vi "Exp Inverse CDF.vi"(9 "b":dbl=3.0, 10 "a":dbl=1.0, 11 "cdf(x)":dbl=0.486583) -> (0 "error":i32, 3 "x":dbl=3.000000695531575)   [LabVIEW 2020, in "NI_Gmath.lvlib"]
doc: "Computes the continuous inverse cumulative distribution function (CDF) of the various distributions. You must manually select the polymorphic instance to use."
uses:
  <vilib>/gmath/NI_Gmath.lvlib
  <vilib>/gmath/statdist.llb/st_error_code.ctl
panel:
  # "Exp Inverse CDF"
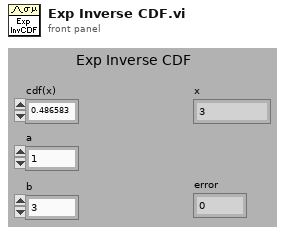
[diagram p1: front panel]
types:
  T1 = typedef "NI_Gmath.lvlib/st_error_code.ctl" = i32
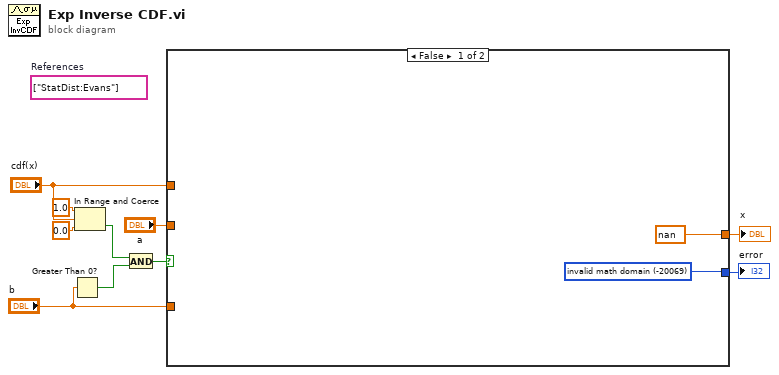
[diagram p0: block diagram]
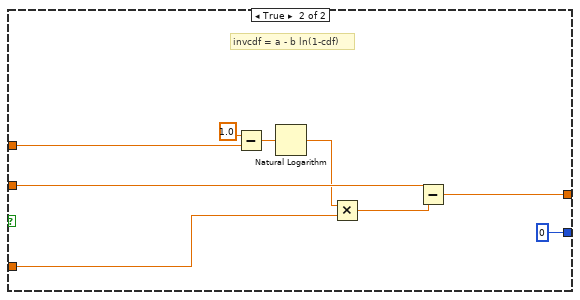
[diagram p2: hidden frame]
diagram:
  (unwired) string[] ["StatDist:Evans"]  # References
  n1 = Greater Than 0?(x="b") -> (x > 0?=w2:bool)
  n2 = In Range and Coerce(upper limit=1.0, x="cdf(x)", lower limit=0.0) -> (In Range?=w1:bool)  [unwired: 1 out]
  n3 = And(x=w1, y=w2) -> (x .and. y?=w3:bool)
  n4 = case shown="False" w3 {
    tunnel: "b" -> [_ w18]
    tunnel: [w11 0 ("invalid math domain")] -> w9
    tunnel: [nan w20] -> w8
    tunnel: "cdf(x)" -> [_ w17]
    tunnel: "a" -> [_ w19]
    frame False {
      w11 = T1 -20069 items=["invalid math domain"=-20069, "Fourier interpolation size m >= n"=-20070, "empty array"=-20003] ("stat interp error code")
    }
    frame True {
      # "invcdf = a - b ln(1-cdf)"
      n5 = Subtract(x=1.0 ("y"), y=w17) -> (x-y=w15:dbl)
      n6 = Natural Logarithm(1:w15) -> (0:w13:dbl)
      n7 = Multiply(x=w13, y=w18) -> (x*y=w14:dbl)
      n8 = Subtract(x=w19, y=w14) -> (x-y=w20:dbl)
    }
  }
  "x" <- w8
  "error" <- w9
